vi "Set Operational Force Test Settings.vi"(10 "Operational Force Test Settings":T1 {"Sample Time (s)" format="%.4f"; "Process Time (s)" format="%.4f"; "Max Moment (NM)" format="%.4f"; "Max Force Error (N)" format="%.4f"}, 11 "Model in":refnum<class "Model.lvclass">) -> (3 "Model out":refnum<class "Model.lvclass">)   [LabVIEW 2016]
uses:
  Model.lvclass
  Typedefs/OperationalForceTestSettings.ctl
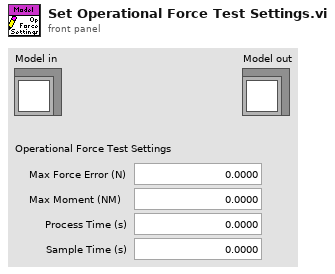
[diagram p1: front panel]
types:
  T1 = typedef "OperationalForceTestSettings.ctl" = cluster{"Max Force Error (N)":dbl, "Max Moment (NM)":dbl, "Process Time (s)":dbl, "Sample Time (s)":dbl}
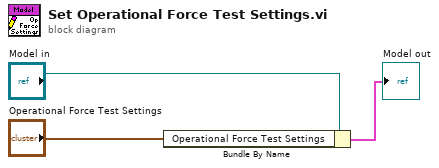
[diagram p0: block diagram]
diagram:
  n1 = Bundle By Name(cluster="Model in", "Operational Force Test Settings"="Operational Force Test Settings") -> (→"Model out":cluster{})
